vi "myRIO_BRig_Host_parse_dataBlock__v2.vi"(10 "input_dataCurrent":u16[](array[numeric]), 11 "input_dataBlock":u16[][](array[numeric])) -> (0 "BlockR_T2R_avg":dbl caption="Trials2Reward", 1 "BlockR_BTPR_avg":dbl caption="BadTrialsPostReward", 2 "BlockL_BTPR_avg":dbl caption="BadTrialsPostReward" format="%#_3g", 3 "BlockL_T2R_avg":dbl caption="Trials2Reward" format="%#_3g", 4 "BlockR_BTPR_cur":u16 caption="BadTrialsPostReward", 5 "BlockL_BTPR_cur":u16 caption="BadTrialsPostReward", 6 "BlockR_T2R_cur":u16 caption="Trials2Reward", 7 "BlockL_T2R_cur":u16 caption="Trials2Reward")   [LabVIEW 2014]
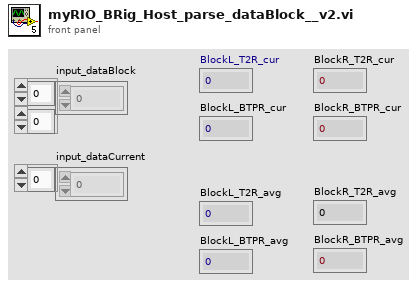
[diagram p1: front panel]
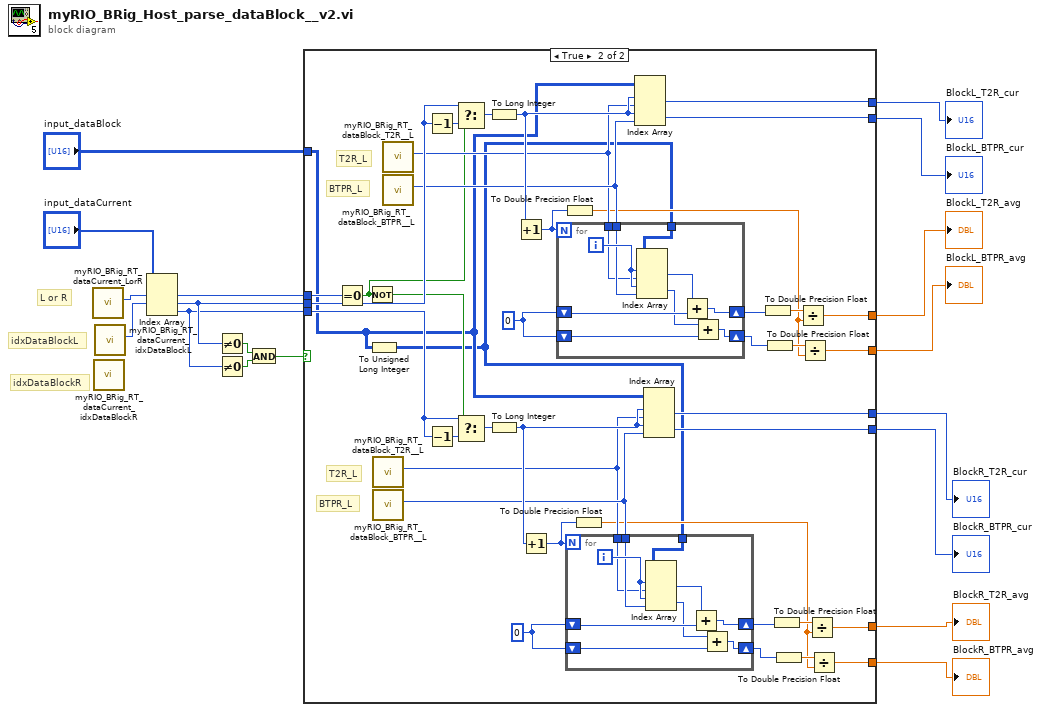
[diagram p0: block diagram]
diagram:
  # "L or R"
  # "idxDataBlockR"
  # "idxDataBlockL"
  n1 = call "myRIO_BRig_RT_dataCurrent_LorR.vi"() -> ("output_LorR"=w16:i32)  [unwired: 11 in]
  n2 = call "myRIO_BRig_RT_dataCurrent_idxDataBlockR.vi"() -> ()  [unwired: 11 in, 1 out]
  n3 = call "myRIO_BRig_RT_dataCurrent_idxDataBlockL.vi"() -> ("output_idxDataBlock__L"=w17:i32)  [unwired: 11 in]
  n4 = Index Array(array="input_dataCurrent", index #1=w16, index #2=w17) -> (element #1=w11:u16, element #2=w10:u16, element #3=w9:u16)  [unwired: 1 in]
  n5 = Not Equal To 0?(x=w10) -> (x != 0?=w14:bool)
  n6 = Not Equal To 0?(x=w9) -> (x != 0?=w15:bool)
  n7 = And(x=w14, y=w15) -> (x .and. y?=w13:bool)
  n8 = case shown="True" w13 {
    tunnel: "input_dataBlock" -> [_ w20]
    tunnel: w11 -> [_ w28]
    tunnel: w10 -> [_ w56]
    tunnel: w9 -> [_ w25]
    tunnel: [_ w54] -> w6
    tunnel: [_ w53] -> w5
    tunnel: [_ w46] -> w8
    tunnel: [_ w41] -> w7
    tunnel: [_ w24] -> w2
    tunnel: [_ w23] -> w1
    tunnel: [_ w22] -> w3
    tunnel: [_ w21] -> w4
    frame False {
    }
    frame True {
      w35 = u32 0
      w49 = u32 0
      # "BTPR_L"
      # "T2R_L"
      # "BTPR_L"
      # "T2R_L"
      n9 = Equal To 0?(x=w28) -> (x = 0?=w27:bool)
      n10 = Not(x=w27) -> (.not. x?=w26:bool)
      n11 = To Unsigned Long Integer(number=w20) -> (unsigned 32bit integer=w19:u32[][])
      n12 = call "myRIO_BRig_RT_dataBlock_T2R__L.vi"() -> ("output_T2R__L"=w36:i32)  [unwired: 11 in]
      n13 = call "myRIO_BRig_RT_dataBlock_BTPR__L.vi"() -> ("output_BTPR__L"=w37:i32)  [unwired: 11 in]
      n14 = call "myRIO_BRig_RT_dataBlock_T2R__L.vi"() -> ("output_T2R__L"=w50:i32)  [unwired: 11 in]
      n15 = call "myRIO_BRig_RT_dataBlock_BTPR__L.vi"() -> ("output_BTPR__L"=w51:i32)  [unwired: 11 in]
      n16 = Decrement(x=w56) -> (x-1=w57:u16)
      n17 = Decrement(x=w25) -> (x-1=w40:u16)
      n18 = Select(t=w56, s=w27, f=w57) -> (s? t:f=w55:u16)
      n19 = Select(t=w25, s=w26, f=w40) -> (s? t:f=w39:u16)
      n20 = To Long Integer(number=w55) -> (32bit integer=w52:i32)
      n21 = To Long Integer(number=w39) -> (32bit integer=w38:i32)
      n22 = Increment(x=w52) -> (x+1=w44:i32)
      n23 = Increment(x=w38) -> (x+1=w31:i32)
      n24 = for {
        N: w44 -> [_]
        tunnel: w51 -> [w76]
        tunnel: w50 -> [w75]
        shift-right: [w71] -> w47
        shift-left: w49 -> [w72]
        shift-right: [w74] -> w42
        shift-left: w49 -> [w73]
        tunnel: w19 -> [w70]
        i -> [w77]
        n25 = Index Array(array=w70, index (row) #1=w77, index (col) #1=w75, index (row) #2=w77, index (col) #2=w76) -> (element #1=w69:u32, element #2=w68:u32)
        n26 = Add(x=w69, y=w72) -> (x+y=w71:u32)
        n27 = Add(x=w68, y=w73) -> (x+y=w74:u32)
      }
      n28 = To Double Precision Float(number=w44) -> (double precision float=w43:dbl)
      n29 = for {
        N: w31 -> [_]
        tunnel: w37 -> [w66]
        tunnel: w36 -> [w65]
        shift-right: [w61] -> w33
        shift-left: w35 -> [w62]
        shift-right: [w64] -> w29
        shift-left: w35 -> [w63]
        tunnel: w19 -> [w60]
        i -> [w67]
        n30 = Index Array(array=w60, index (row) #1=w67, index (col) #1=w65, index (row) #2=w67, index (col) #2=w66) -> (element #1=w58:u32, element #2=w59:u32)
        n31 = Add(x=w58, y=w62) -> (x+y=w61:u32)
        n32 = Add(x=w59, y=w63) -> (x+y=w64:u32)
      }
      n33 = To Double Precision Float(number=w31) -> (double precision float=w30:dbl)
      n34 = Index Array(array=w20, index (row) #1=w52, index (col) #1=w50, index (row) #2=w52, index (col) #2=w51) -> (element #1=w54:u16, element #2=w53:u16)
      n35 = Index Array(array=w20, index (row) #1=w38, index (col) #1=w36, index (row) #2=w38, index (col) #2=w37) -> (element #1=w24:u16, element #2=w23:u16)
      n36 = To Double Precision Float(number=w47) -> (double precision float=w48:dbl)
      n37 = To Double Precision Float(number=w42) -> (double precision float=w45:dbl)
      n38 = To Double Precision Float(number=w33) -> (double precision float=w34:dbl)
      n39 = To Double Precision Float(number=w29) -> (double precision float=w32:dbl)
      n40 = Divide(x=w48, y=w43) -> (x/y=w46:dbl)
      n41 = Divide(x=w45, y=w43) -> (x/y=w41:dbl)
      n42 = Divide(x=w34, y=w30) -> (x/y=w21:dbl)
      n43 = Divide(x=w32, y=w30) -> (x/y=w22:dbl)
    }
  }
  "BlockR_T2R_avg" <- w4
  "BlockR_BTPR_avg" <- w3
  "BlockR_T2R_cur" <- w2
  "BlockR_BTPR_cur" <- w1
  "BlockL_T2R_avg" <- w8
  "BlockL_BTPR_avg" <- w7
  "BlockL_T2R_cur" <- w6
  "BlockL_BTPR_cur" <- w5
